vi "TimeTag_Sept_2022.vi"() -> ()   [LabVIEW 2015]
doc: "This sample project is built upon the standard state machine template and shows how you could create an application that acquires, analyzes, and presents data. It includes functionality for presenting configuration dialogs, preserving settings between executions, loading and saving data, as well as exporting graph images and text files.\n\nIt is most appropriate for data that is acquired instantly as it does not allow for screen updates mid acquisition nor does it allow for continuous streaming to disk."
uses:
  <vilib>/ptbypt/NI_PtbyPt.lvlib
panel:
  out "Ch4 100sec avg":dbl
  out "Ch2 100 sec avg":dbl
  out "real coin cps 100 pt\n avg":dbl
  out "all coin cps":dbl
  out "real coin cps":dbl
  out "random coin cps":dbl
  out "Real coin cps":dbl(graph)
  out "total coin/sec - total random coin/sec":dbl
  out "total random coincidences/sec":dbl
  out "Total Coin per sec":dbl
  out "Ch2/4 coin/sec":dbl(graph)
  out "Ch2/4 Total Coincidences":dbl
  out "Channel 2 CPS":dbl(graph)
  out "Channel 4 CPS":dbl(graph)
  out "Total Ch2 CPS":dbl
  out "Total Ch4 CPS":dbl
  in  "Averaging":dbl=10.0
  in  "Runs":dbl=100.0
  in  "Pulse TTL 2":bool
  in  "Pulse TTL 1":bool
  in  "Toggle\nTTL 2":bool
  in  "Toggle\nTTL 1":bool
  out "Total Starts":dbl
  in  "Record data":bool
  out "Initial time":dbl
  out "Elapsed time (s)":dbl
  out "FPGA_Run Status":dbl
  out "USB_Open Status":dbl
  out "Channel 4 Total\nCounts":dbl
  out "Channel 3 Total\nCounts":dbl
  out "Channel 2 Total\nCounts":dbl
  out "Channel 1 Total\nCounts":dbl
  in  "File Name":string="C:\\FPGA\\test.txt"
  out "?":dbl
  out "?":dbl
  out "?":dbl
  out "?":dbl
  out "stats":i64[](array[numeric])
  in  "Stop":bool
  out "Channel 4 CPS":dbl(knob) scale=0.0..2000000.0
  out "Channel 3 CPS":dbl(knob) scale=0.0..600.0
  out "Channel 2 CPS":dbl(knob) scale=0.0..700.0
  out "Channel 1 CPS":dbl(knob) scale=0.0..600.0
  # "Starts"
  # "Channel 1"
  # "Channel 2"
  # "Channel 3"
  # "Channel 4"
  # "Coincidence Channels 1 & 2"
  # "Coincidence Channels 1 & 3"
  # "Coincidence Channels 1 & 4"
  # "Coincidence Channels 2 & 3"
  # "Coincidence Channels 2 & 4"
  # "Coincidence Channels 3 & 4"
  # "Coincidence Channels 1 & 2 & 3"
  # "Coincidence Channels 1 & 2 & 4"
  # "Coincidence Channels 1 & 3 & 4"
  # "Coincidence Channels 2 & 3 & 4"
  # "C:\\FPGA_Lauren"
  # "Coincidence Channels 1 & 2 & 3 & 4"
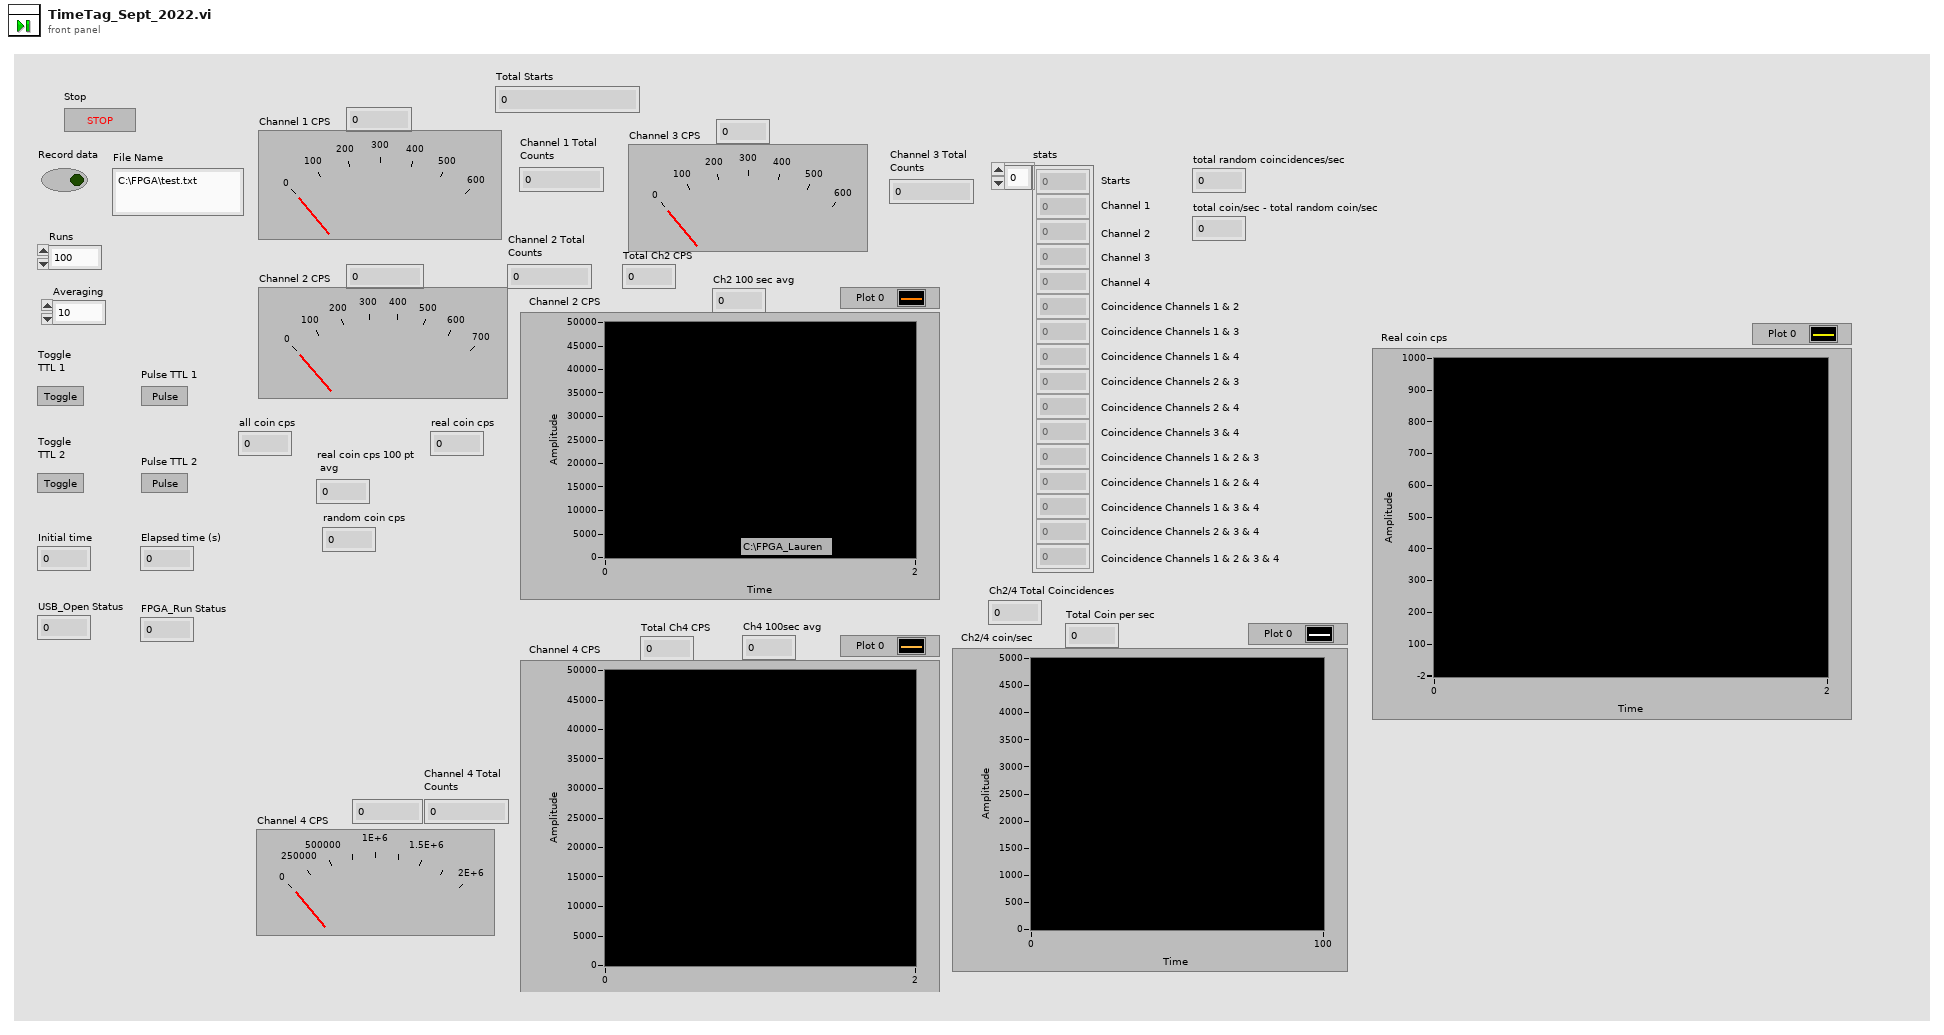
[diagram p1: front panel]
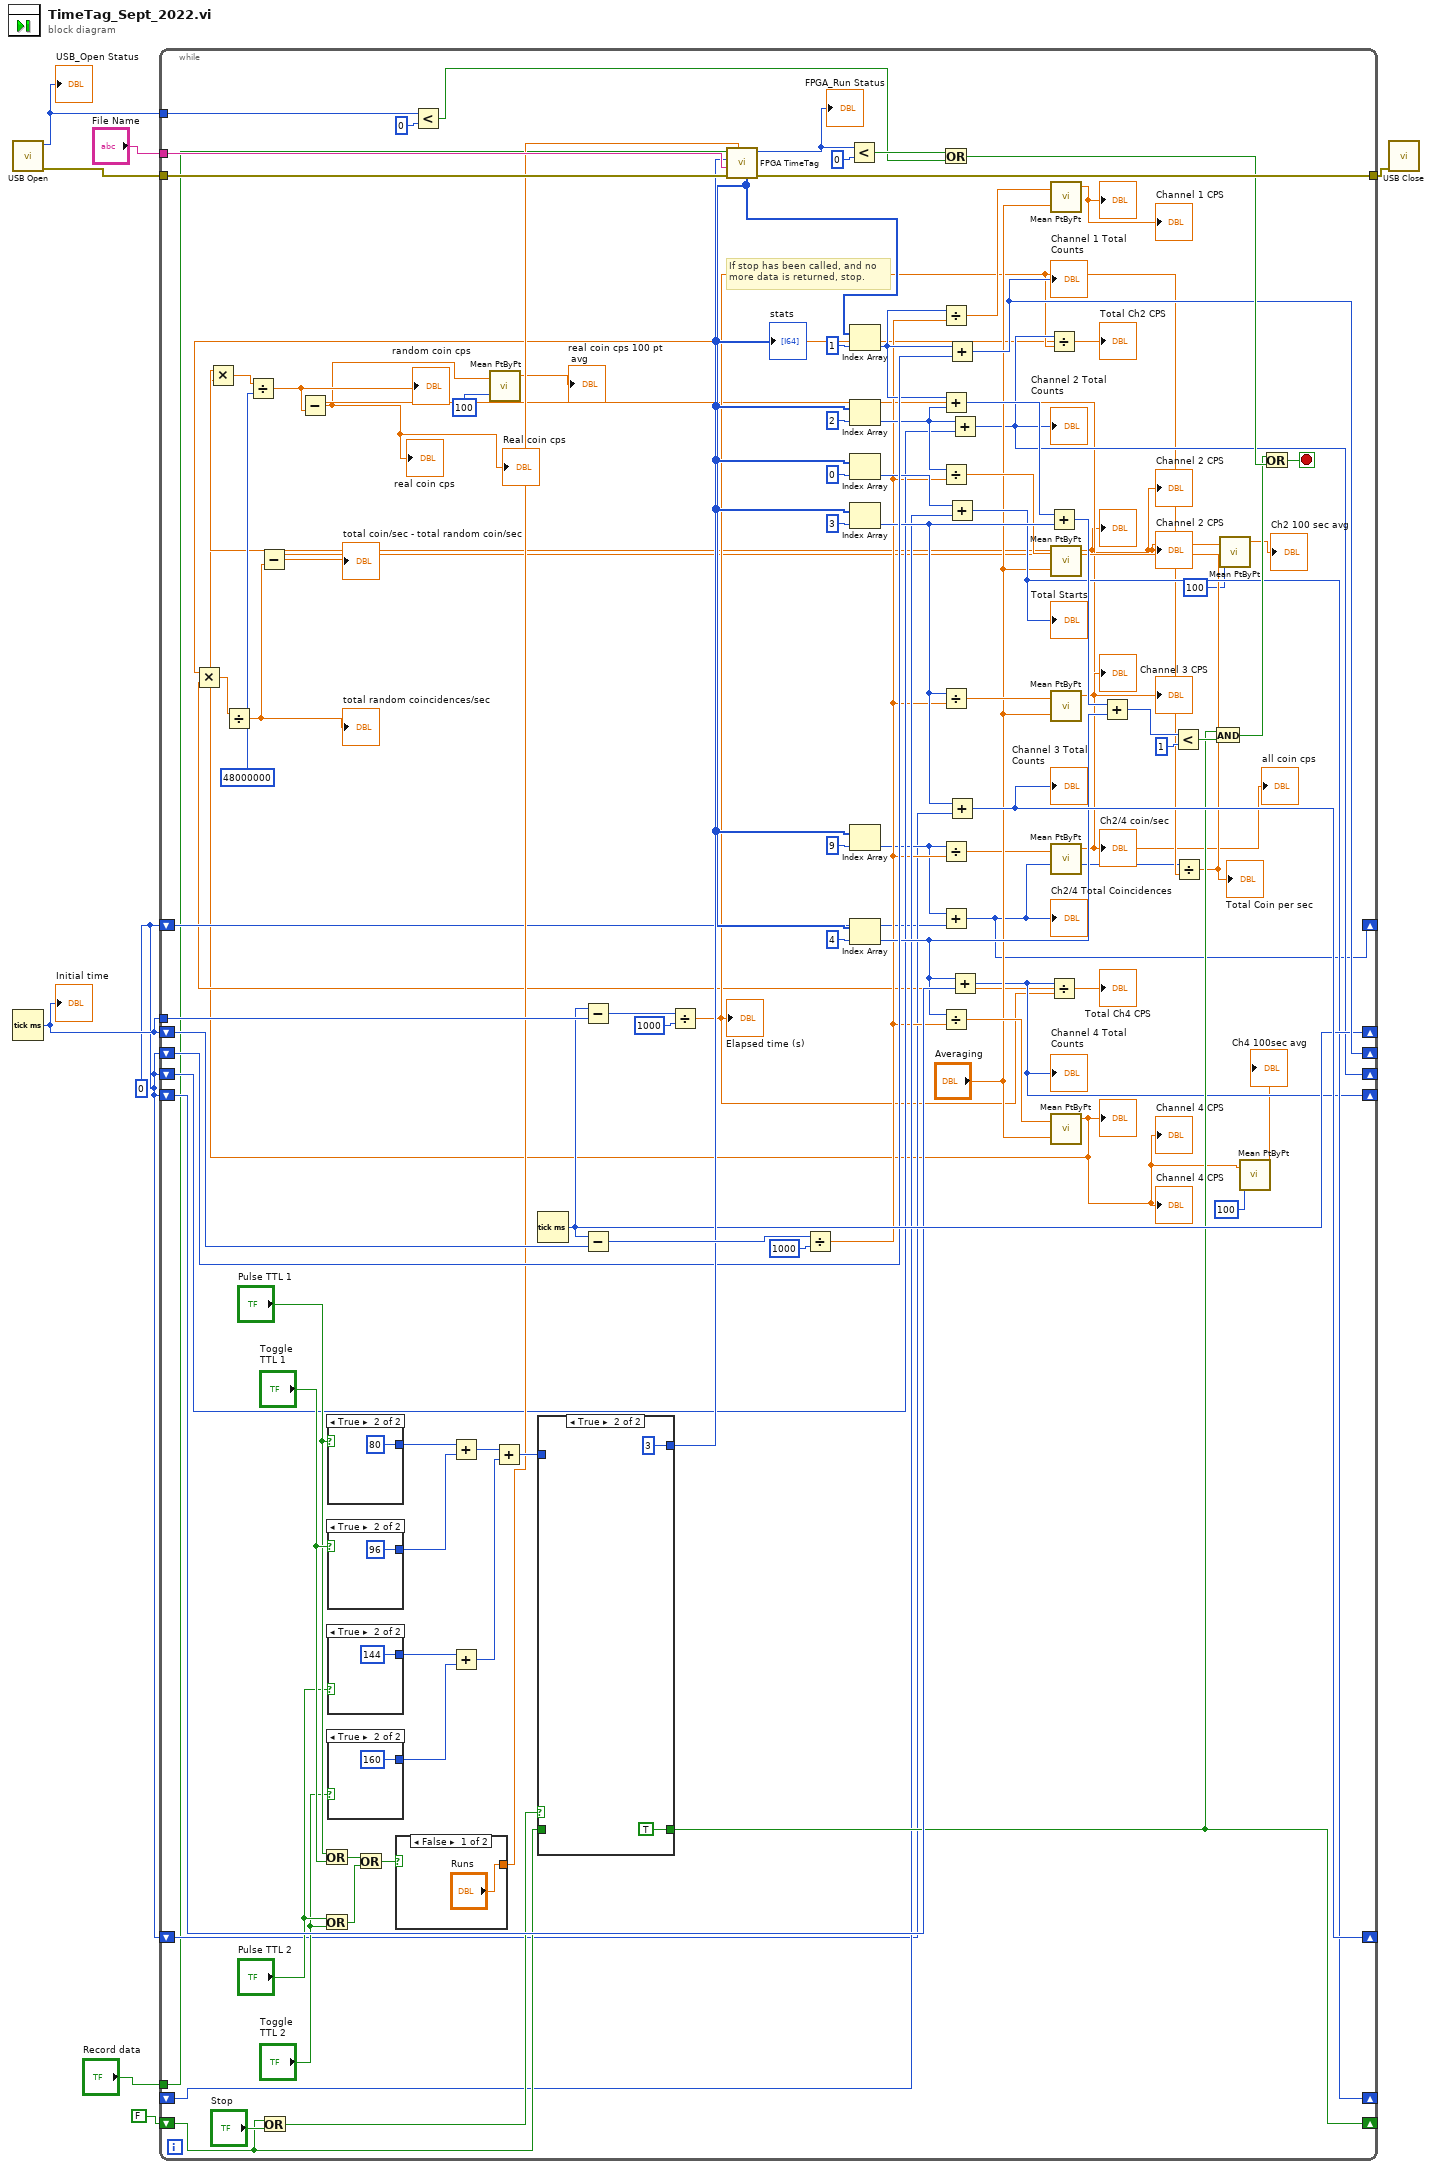
[diagram p0: block diagram]
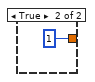
[diagram p2: hidden frame]
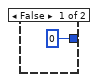
[diagram p3: hidden frame]
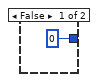
[diagram p4: hidden frame]
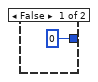
[diagram p5: hidden frame]
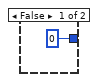
[diagram p6: hidden frame]
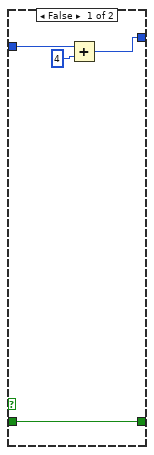
[diagram p7: hidden frame]
diagram:
  w1 = 0
  n1 = call "USB Open.vi"() -> ("error out"=w6:errorcluster, "function return"=w3:i32)  [unwired: 10 in]
  "USB_Open Status" <- w3
  n2 = Tick Count (ms)() -> (millisecond timer value=w4:u32)
  "Initial time" <- w4
  n3 = while {
    tunnel: w4 -> [w107]
    shift-right: [w86] -> _
    shift-left: w1 -> [w82]
    shift-right: [w40] -> _
    shift-left: w1 -> [w36]
    shift-right: [w85] -> _
    shift-left: w1 -> [w32]
    shift-right: [w41] -> _
    shift-left: w1 -> [w81]
    tunnel: w6 -> [w97]
    tunnel: [w98] -> w5
    tunnel: "Record data" -> [w10]
    tunnel: "File Name" -> [w96]
    shift-right: [w83] -> _
    shift-left: w4 -> [w94]
    tunnel: w3 -> [w90]
    shift-right: [w70] -> _
    shift-left: FALSE -> [w67]
    shift-right: [w63] -> _
    shift-left: _ -> [w64]
    shift-right: [w29] -> _
    shift-left: w1 -> [w31]
    stop <- w99 stop-if-true
    w23 = 48000000
    # "If stop has been called, and no\nmore data is returned, stop."
    n4 = Or(x=w67, y="Stop") -> (x .or. y?=w69:bool)
    n5 = Or(x="Pulse TTL 1", y="Toggle\nTTL 1") -> (x .or. y?=w54:bool)
    n6 = Or(x="Pulse TTL 2", y="Toggle\nTTL 2") -> (x .or. y?=w55:bool)
    n7 = case shown="True" "Pulse TTL 1" {
      tunnel: [0 80] -> w62
      frame False {
      }
      frame True {
      }
    }
    n8 = case shown="True" "Toggle\nTTL 1" {
      tunnel: [0 96] -> w61
      frame False {
      }
      frame True {
      }
    }
    n9 = case shown="True" "Pulse TTL 2" {
      tunnel: [0 144] -> w58
      frame False {
      }
      frame True {
      }
    }
    n10 = case shown="True" "Toggle\nTTL 2" {
      tunnel: [0 160] -> w59
      frame False {
      }
      frame True {
      }
    }
    n11 = Or(x=w54, y=w55) -> (x .or. y?=w56:bool)
    n12 = case shown="False" w56 {
      tunnel: ["Runs" 1] -> w52
      frame False {
      }
      frame True {
      }
    }
    n13 = Less?(x=w90, y=0) -> (x < y?=w88:bool)
    n14 = Add(x=w62, y=w61) -> (x+y=w60:i32)
    n15 = Add(x=w58, y=w59) -> (x+y=w57:i32)
    n16 = Add(x=w60, y=w57) -> (x+y=w53:i32)
    n17 = Tick Count (ms)() -> (millisecond timer value=w83:u32)
    n18 = case shown="True" w69 {
      tunnel: [w119 3] -> w84
      tunnel: [w121 TRUE] -> w70
      tunnel: w67 -> [w121 _]
      tunnel: w53 -> [w118 _]
      frame False {
        n19 = Add(x=w118, y=4) -> (x+y=w119:i32)
      }
      frame True {
      }
    }
    n20 = Subtract(x=w83, y=w107) -> (x-y=w106:u32)
    n21 = Subtract(x=w83, y=w94) -> (x-y=w93:u32)
    n22 = Divide(x=w106, y=1000) -> (x/y=w30:dbl)
    "Elapsed time (s)" <- w30
    n23 = call "FPGA TimeTag.vi"("runs"=w52, "error in (no error)"=w97, "fileName"=w96, "fpgaCommand"=w84, "saveData"=w10) -> ("error out"=w98:errorcluster, "function return"=w95:i32, "stats"=w38:i64[])  [unwired: 4 in]
    "stats" <- w38
    "FPGA_Run Status" <- w95
    n24 = Divide(x=w93, y=1000) -> (x/y=w35:dbl)
    n25 = Less?(x=w95, y=0) -> (x < y?=w89:bool)
    n26 = Index Array(array=w38, index=1) -> (element=w73:i64)
    n27 = Index Array(array=w38, index=2) -> (element=w80:i64)
    n28 = Index Array(array=w38, index=0) -> (element=w65:i64)
    n29 = Index Array(array=w38, index=3) -> (element=w76:i64)
    n30 = Index Array(array=w38, index=9) -> (element=w33:i64)
    n31 = Index Array(array=w38, index=4) -> (element=w77:i64)
    n32 = Or(x=w89, y=w88) -> (x .or. y?=w87:bool)
    n33 = Divide(x=w73, y=w35) -> (x/y=w47:dbl)
    n34 = Add(x=w73, y=w80) -> (x+y=w75:i64)
    n35 = Divide(x=w80, y=w35) -> (x/y=w46:dbl)
    n36 = Divide(x=w76, y=w35) -> (x/y=w45:dbl)
    n37 = Divide(x=w33, y=w35) -> (x/y=w34:dbl)
    n38 = Add(x=w33, y=w31) -> (x+y=w29:i64)
    "Ch2/4 Total Coincidences" <- w29
    n39 = Divide(x=w77, y=w35) -> (x/y=w43:dbl)
    n40 = Add(x=w73, y=w82) -> (x+y=w86:i64)
    "Channel 1 Total\nCounts" <- w86
    n41 = Add(x=w65, y=w64) -> (x+y=w63:i64)
    "Total Starts" <- w63
    n42 = Add(x=w76, y=w32) -> (x+y=w85:i64)
    "Channel 3 Total\nCounts" <- w85
    n43 = Add(x=w80, y=w36) -> (x+y=w40:i64)
    "Channel 2 Total\nCounts" <- w40
    n44 = Add(x=w77, y=w81) -> (x+y=w41:i64)
    "Channel 4 Total\nCounts" <- w41
    n45 = Divide(x=w40, y=w30) -> (x/y=w26:dbl)
    "Total Ch2 CPS" <- w26
    n46 = Add(x=w75, y=w76) -> (x+y=w79:i64)
    n47 = Divide(x=w41, y=w30) -> (x/y=w25:dbl)
    "Total Ch4 CPS" <- w25
    n48 = Multiply(x=w26, y=w25) -> (x*y=w24:dbl)
    n49 = Divide(x=w24, y=w23) -> (x/y=w27:dbl)
    "total random coincidences/sec" <- w27
    n50 = call <vilib>:"Mean PtByPt.vi"("x"=w47, "sample length"="Averaging") -> ("mean"=→"Channel 1 CPS" →"?":dbl)  [unwired: 2 in, 1 out]
    n51 = call <vilib>:"Mean PtByPt.vi"("x"=w46, "sample length"="Averaging") -> ("mean"=w16:dbl)  [unwired: 2 in, 1 out]
    "Channel 2 CPS" <- w16
    "?" <- w16
    "Channel 2 CPS" <- w16
    n52 = call <vilib>:"Mean PtByPt.vi"("x"=w45, "sample length"="Averaging") -> ("mean"=→"Channel 3 CPS" →"?":dbl)  [unwired: 2 in, 1 out]
    n53 = call <vilib>:"Mean PtByPt.vi"("x"=w34) -> ("mean"=w19:dbl)  [unwired: 3 in, 1 out]
    "Ch2/4 coin/sec" <- w19
    "all coin cps" <- w19
    n54 = call <vilib>:"Mean PtByPt.vi"("x"=w43, "sample length"="Averaging") -> ("mean"=w13:dbl)  [unwired: 2 in, 1 out]
    "Channel 4 CPS" <- w13
    "?" <- w13
    "Channel 4 CPS" <- w13
    n55 = Multiply(x=w16, y=w13) -> (x*y=w22:dbl)
    n56 = Divide(x=w22, y=w23) -> (x/y=w21:dbl)
    "random coin cps" <- w21
    n57 = Subtract(x=w19, y=w21) -> (x-y=w9:dbl)
    "Real coin cps" <- w9
    "real coin cps" <- w9
    n58 = call <vilib>:"Mean PtByPt.vi"("x"=w9, "sample length"=100) -> ("mean"=→"real coin cps 100 pt\n avg":dbl)  [unwired: 2 in, 1 out]
    n59 = Add(x=w79, y=w77) -> (x+y=w78:i64)
    n60 = Less?(x=w78, y=1) -> (x < y?=w72:bool)
    n61 = Divide(x=w29, y=w30) -> (x/y=w28:dbl)
    "Total Coin per sec" <- w28
    n62 = Subtract(x=w28, y=w27) -> (x-y=→"total coin/sec - total random coin/sec":dbl)
    n63 = And(x=w70, y=w72) -> (x .and. y?=w71:bool)
    n64 = call <vilib>:"Mean PtByPt.vi"("x"=w16, "sample length"=100) -> ("mean"=→"Ch2 100 sec avg":dbl)  [unwired: 2 in, 1 out]
    n65 = call <vilib>:"Mean PtByPt.vi"("x"=w13, "sample length"=100) -> ("mean"=→"Ch4 100sec avg":dbl)  [unwired: 2 in, 1 out]
    n66 = Or(x=w71, y=w87) -> (x .or. y?=w99:bool)
  }
  n67 = call "USB Close.vi"("error in (no error)"=w5) -> ()  [unwired: 9 in, 2 out]
